vi "ReadExecutableConfiguration.vi"(8 "Error In":errorcluster, 11 "VI Path":path) -> (0 "Error Out":errorcluster, 1 "Center on Monitor?":bool, 2 "Default Monitor":i32, 3 "Executable Configuration":T1)   [LabVIEW 2013]
uses:
  ExecutableConfiguration.ctl
  <vilib>/Utility/config.llb/Read Key (I32).vi
  <vilib>/Utility/config.llb/Read Key (Boolean).vi
  <vilib>/Utility/config.llb/Read Key (U32).vi
  <vilib>/Utility/config.llb/Read Key (Path).vi
  libs/LV-Utilities/LV-Utilities.lvlib
  <vilib>/Utility/config.llb/NI_LVConfig.lvlib
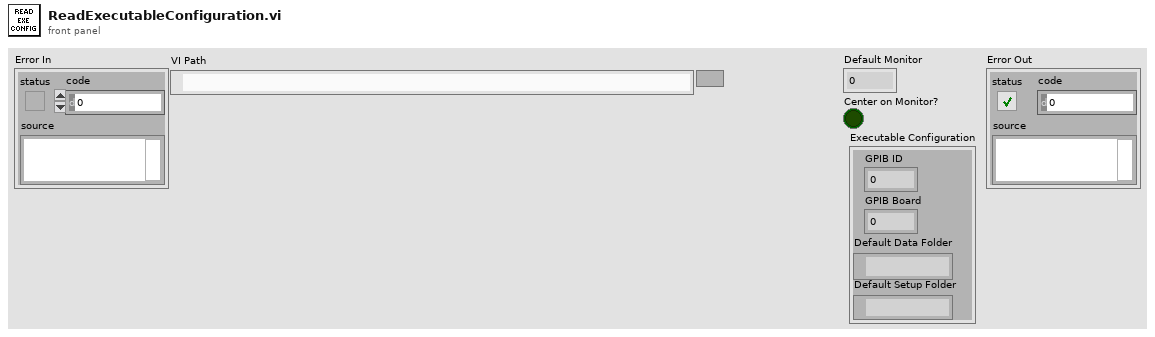
[diagram p1: front panel]
types:
  T1 = typedef "ExecutableConfiguration.ctl" = cluster{"GPIB ID":u8, "GPIB Board":u8, "Default Data Folder":path, "Default Setup Folder":path}
  T2 = typedef "NI_LVConfig.lvlib/Config Data RefNum.ctl" = refnum<k1>
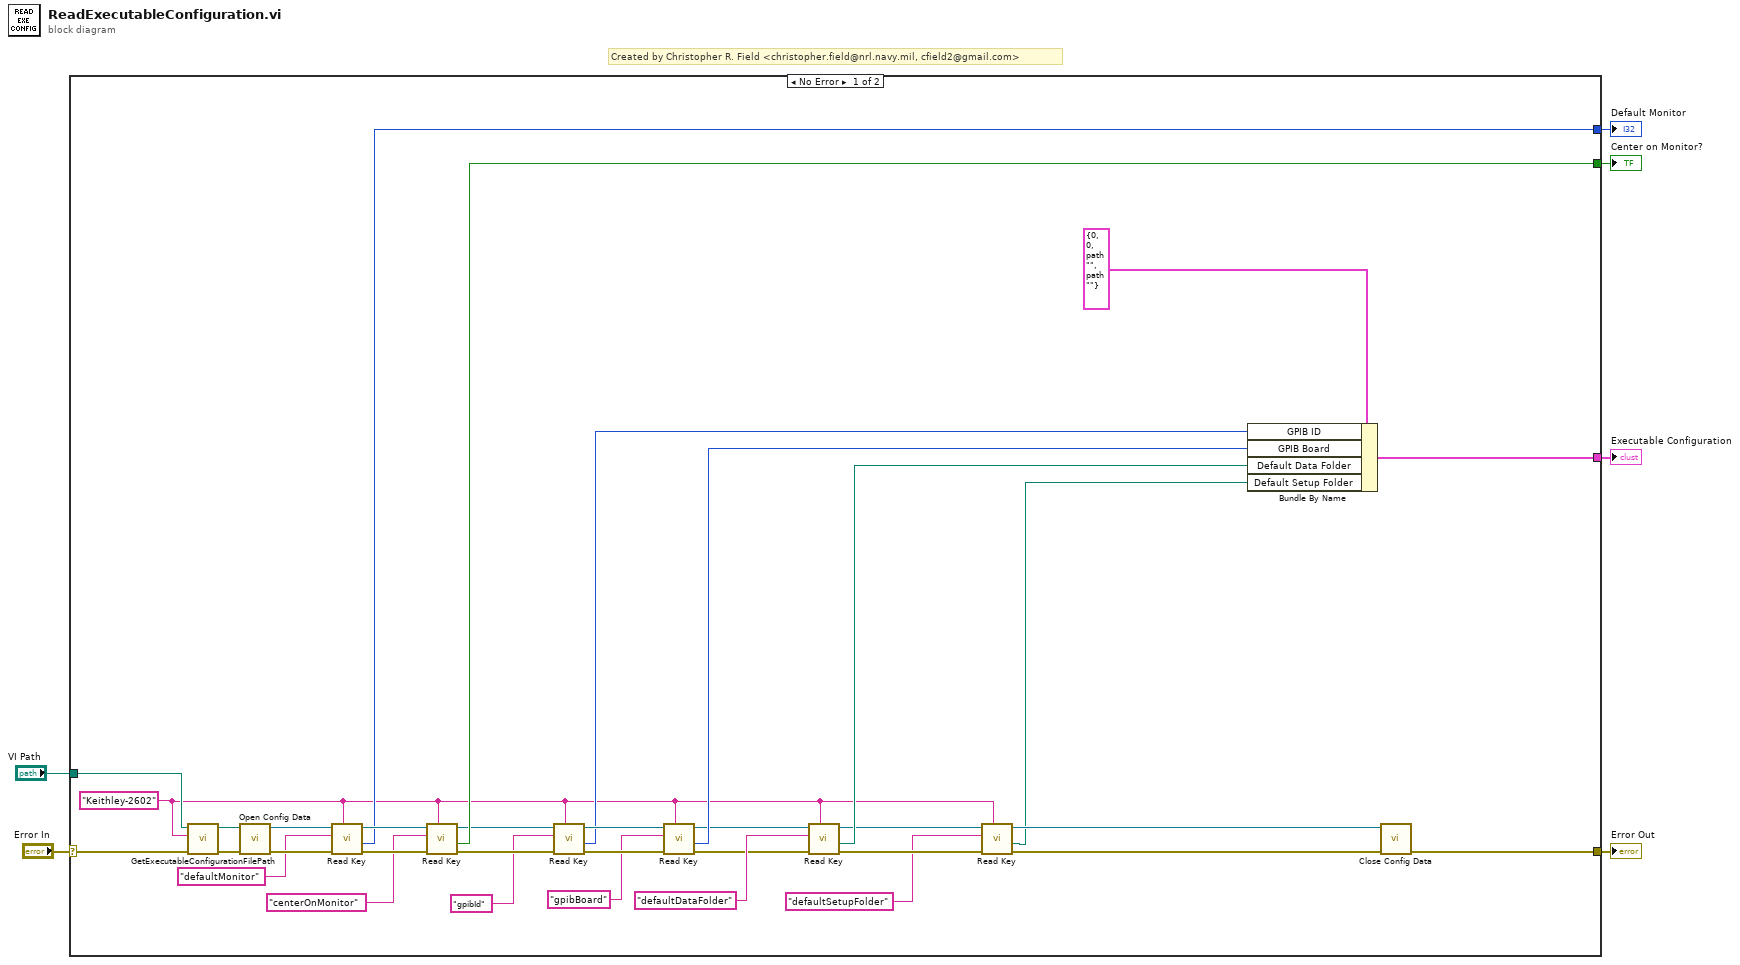
[diagram p0: block diagram]
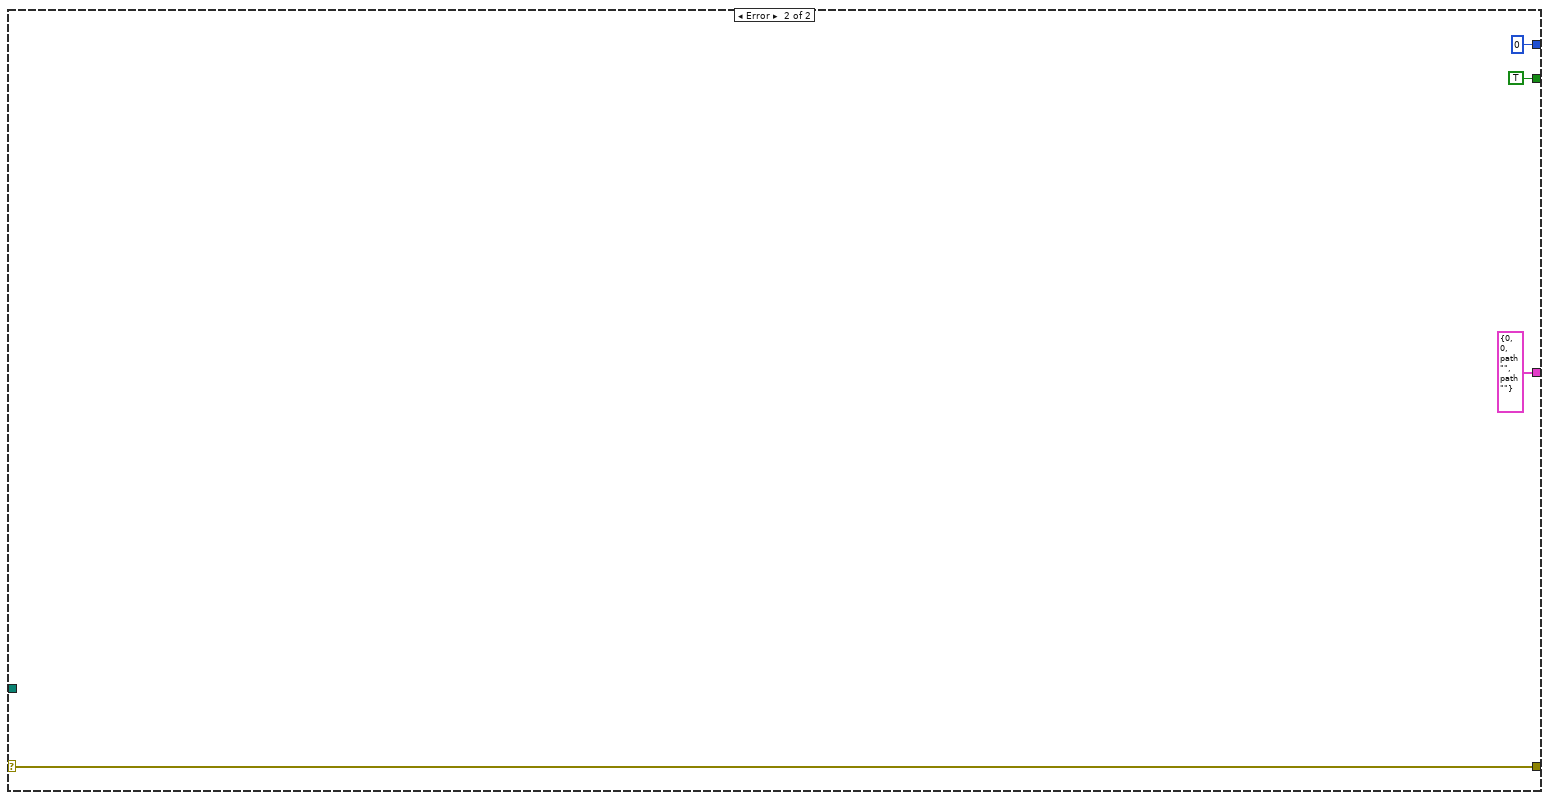
[diagram p2: hidden frame]
diagram:
  # "Created by Christopher R. Field <christopher.field@nrl.navy.mil, cfield2@gmail.com>"
  n1 = case shown="No Error" "Error In" {
    selector: "Error In" -> [w39 w44]
    tunnel: "VI Path" -> [w40 _]
    tunnel: [w31 0 ("value")] -> w4
    tunnel: [w30 TRUE ("value")] -> w3
    tunnel: [w18 T1 {"GPIB ID"=0, "GPIB Board"=0, "Default Data Folder"=path "", "Default Setup Folder"=path ""} ("Executable Configuration")] -> w2
    tunnel: [w17 w44] -> w1
    frame No Error {
      w13 = "Keithley-2602" ("Application Name")
      n2 = call "GetExecutableConfigurationFilePath.vi"("Error In"=w39, "Application Name"=w13, "VI Path"=w40) -> ("Error Out"=w38:errorcluster, "Executable Config File Path"=w7:path)  [unwired: 7 in]
      n3 = call <vilib>:"Open Config Data.vi"("error in (no error)"=w38, "configuration file path"=w7) -> ("error out"=w36:errorcluster, "refnum"=w37:T2)  [unwired: 7 in, 1 out]
      n4 = call-poly <vilib>:"Read Key.vi"("section"=w13, "error in (no error)"=w36, "key"="defaultMonitor", "refnum"=w37) -> ("error out"=w33:errorcluster, "value"=w31:i32, "refnum out"=w34:T2)  [unwired: 4 in, 1 out]
      n5 = call-poly <vilib>:"Read Key.vi"("section"=w13, "error in (no error)"=w33, "key"="centerOnMonitor", "refnum"=w34) -> ("error out"=w28:errorcluster, "value"=w30:bool, "refnum out"=w29:T2)  [unwired: 4 in, 1 out]
      n6 = call-poly <vilib>:"Read Key.vi"("section"=w13, "error in (no error)"=w28, "key"="gpibId", "refnum"=w29) -> ("error out"=w26:errorcluster, "value"=w21:u32, "refnum out"=w27:T2)  [unwired: 4 in, 1 out]
      n7 = call-poly <vilib>:"Read Key.vi"("section"=w13, "error in (no error)"=w26, "key"="gpibBoard", "refnum"=w27) -> ("error out"=w15:errorcluster, "value"=w20:u32, "refnum out"=w16:T2)  [unwired: 4 in, 1 out]
      n8 = call-poly <vilib>:"Read Key.vi"("section"=w13, "error in (no error)"=w15, "key"="defaultDataFolder", "refnum"=w16) -> ("error out"=w12:errorcluster, "value"=w19:path, "refnum out"=w14:T2)  [unwired: 4 in, 1 out]
      n9 = call-poly <vilib>:"Read Key.vi"("section"=w13, "error in (no error)"=w12, "key"="defaultSetupFolder", "refnum"=w14) -> ("error out"=w11:errorcluster, "value"=w9:path, "refnum out"=w10:T2)  [unwired: 4 in, 1 out]
      n10 = Bundle By Name(cluster=T1 {"GPIB ID"=0, "GPIB Board"=0, "Default Data Folder"=path "", "Default Setup Folder"=path ""} ("Executable Configuration"), "GPIB ID"=w21, "GPIB Board"=w20, "Default Data Folder"=w19, "Default Setup Folder"=w9) -> (w18:T1)
      n11 = call <vilib>:"Close Config Data.vi"("error in (no error)"=w11, "refnum"=w10) -> ("error out"=w17:errorcluster)  [unwired: 8 in, 1 out]
    }
    frame Error {
    }
  }
  "Default Monitor" <- w4
  "Center on Monitor?" <- w3
  "Executable Configuration" <- w2
  "Error Out" <- w1
